vi "To Variant.vi"(8 "Error In":errorcluster, 11 "Tree Data":refnum<class "Tree Data.lvclass">) -> (0 "Error Out":errorcluster, 3 "Variant":variant)   [LabVIEW 2020, in "NI_VIAnCFGDataStructure.lvlib" / "Tree.lvclass"]
doc: "Converts the Tree Data type into LV Variant data.\n\nTo support more type you need to create your own conversion method using LabVIEW Data Type Parsing API. Use this method as an example."
uses:
  <vilib>/addons/analyzer/VIAnCFGDataStructure/Tree Manager/Tree.lvclass
  <vilib>/addons/analyzer/VIAnCFGDataStructure/Tree Data/Tree Data.lvclass
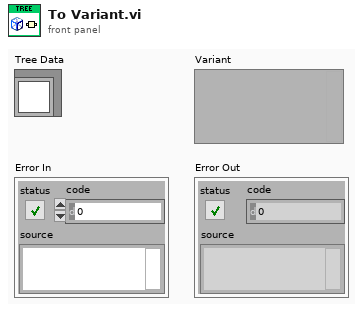
[diagram p1: front panel]
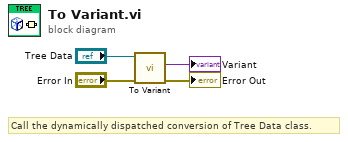
[diagram p0: block diagram]
diagram:
  # "Call the dynamically dispatched conversion of Tree Data class."
  n1 = call-dynamic "To Variant.vi"("Error In"="Error In", "Tree Data"="Tree Data") -> ("Error Out"=→"Error Out":errorcluster, "Variant"=→"Variant":variant)  [unwired: 8 in]
